vi "ControlRelay_ver10.vi"(0 "VISA session":refnum<visa-resource-name>="COM3", 1 "baud rate (9600)":u32=9600, 2 "data bits (8)":u16=8, 3 "stop bits (10: 1 bit)":u16(ring)=10 items=["1.0"=10, "1.5"=15, "2.0"=20], 4 "parity (0:none)":enum16{"None", "Odd", "Even", "Mark", "Space"}(ring), 5 "error in (no error)":errorcluster {"code" format="%.0x"}, 6 "BoardSelection":enum32{"Board A", "Board B"}(radio), 7 "Return Byte":u32=4, 8 "BoardA":T1(ring), 9 "flow control (0:none)":u16(ring) items=["None", "XON/XOFF", "RTS/CTS", "XON/XOFF & RTS/CTS", "DTR/DSR", "XON/XOFF & DTR/DSR"], 10 "BoardB":T2(ring), 11 "write buffer":string="Zc", 12 "Relay Setting":T3(radio)) -> (14 "Status of Set CMD":bool, 15 "ReturnCMD":string, 18 "Status of Manual CMD":bool, 19 "error out":errorcluster {"code" format="%.0x"})   [LabVIEW 2011]
uses:
  <vilib>/Instr/_visa.llb/VISA Configure Serial Port (Instr).vi
panel:
  out "read buffer 2":string
  out "after substring":string
  out "before substring":string
  out "TestPlanOutA":string caption="TestPlan on Board A"
  out "TestPlanOutB":string caption="TestPlan on Board B"
  in  "BoardB_TestPlan":T4(ring)
  in  "BoardA_TestPlan":T5(ring)
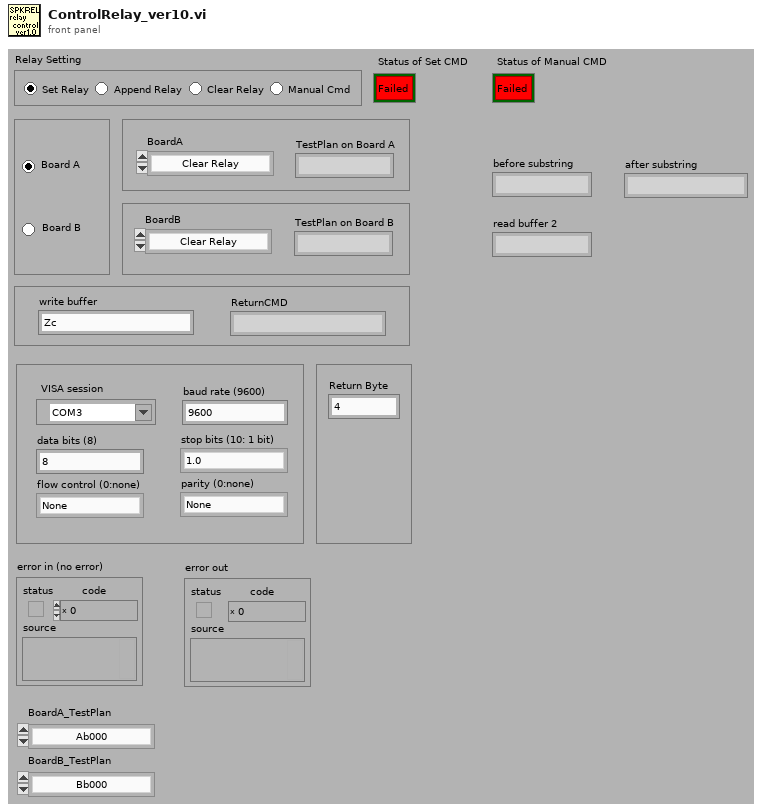
[diagram p1: front panel]
types:
  T1 = enum16{"Clear Relay", "Move Fixture in", "Move Fixture out", "Press UUT", "Press micro SW ", "Probe location M1", "Initial test 1", "Initial test 2", "Initial test 3", "Initial test 4", "Initial test 5", "Initial test 6", "Initial test 7", "Initial test 8", "Initial test 9", "Initial test 10", "Power on UUT", "Test of service pin", "Test of I2C Reset", "Test of I2C Address", "Test of I2C SDA", "Test of I2C SCK"}
  T2 = enum16{"Clear Relay", "Verify Fixture", "Connect RS 232 to UUT", "Test of CD Sinking", "Test of CTS Sinking", "Test of DTR Sinking", "Test of RTS", "Test of DSR", "Test of Lon bus (EKC204A1)", "Test of Lon bus CPU (SM Dummy )", "Test of RS485 (EKC204A2)", "Test of LAN Interface"}
  T3 = enum32{"Set Relay", "Append Relay", "Clear Relay", "Manual Cmd"}
  T4 = enum16{"Bb000", "Bb001", "Bb002", "Bb003", "Bb004", "Bb005", "Bb006", "Bb007", "Bb008", "Bb009", "Bb010", "Bb011"}
  T5 = enum16{"Ab000", "Ab001", "Ab002", "Ab003", "Ab004", "Ab005", "Ab006", "Ab007", "Ab008", "Ab009", "Ab010", "Ab011", "Ab012", "Ab013", "Ab014", "Ab015", "Ab016", "Ab017", "Ab018", "Ab019", "Ab020", "Ab021"}
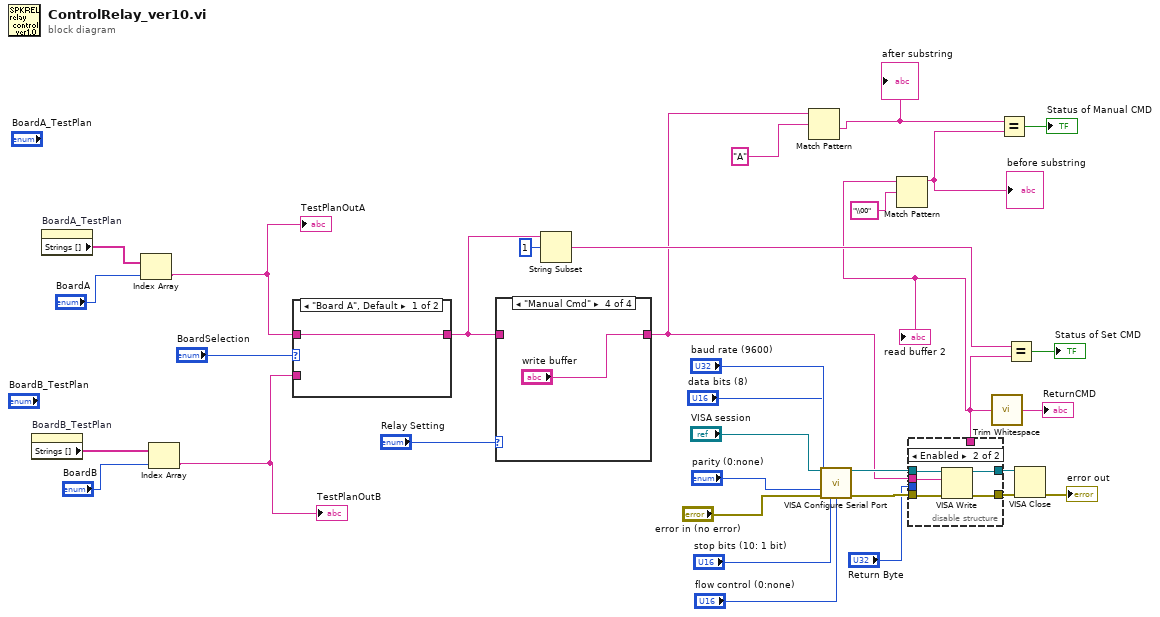
[diagram p0: block diagram]
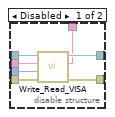
[diagram p2: hidden frame]
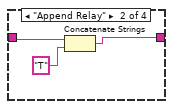
[diagram p4: hidden frame]
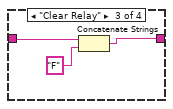
[diagram p5: hidden frame]
diagram:
  n1 = property on="BoardB_TestPlan" class="Enum (strict)"() -> ("Strings []"=w30:string[])  [unwired: 2 in, 2 out]
  n2 = property on="BoardA_TestPlan" class="Enum (strict)"() -> ("Strings []"=w31:string[])  [unwired: 2 in, 2 out]
  n3 = Index Array(array=w31, index="BoardA") -> (element=w8:string)
  "TestPlanOutA" <- w8
  n4 = Index Array(array=w30, index="BoardB") -> (element=w9:string)
  "TestPlanOutB" <- w9
  n5 = case shown="\"Board A\", Default" "BoardSelection" {
    tunnel: w8 -> [w34 _]
    tunnel: [w34 w35] -> w14
    tunnel: w9 -> [_ w35]
    frame "Board A", Default {
    }
    frame "Board B" {
    }
  }
  n6 = case shown="\"Manual Cmd\"" "Relay Setting" {
    tunnel: w14 -> [w36 w39 w41 _]
    tunnel: [w36 w38 w40 "write buffer"] -> w6
    frame "Set Relay", Default {
    }
    frame "Append Relay" {
      n7 = Concatenate Strings(w39, "T" ("string")) -> (w38:string)
    }
    frame "Clear Relay" {
      n8 = Concatenate Strings(w41, "F" ("string")) -> (w40:string)
    }
    frame "Manual Cmd" {
    }
  }
  n9 = String Subset(string=w14, offset (0)=1) -> (substring=w12:string)  [unwired: 1 out]
  n10 = Match Pattern(string=w6, regular expression="A") -> (after substring=w4:string)  [unwired: 4 out]
  "after substring" <- w4
  n11 = call-poly "VISA Configure Serial Port"("VISA resource name"="VISA session", "baud rate (9600)"="baud rate (9600)", "data bits (8)"="data bits (8)", "parity (0:none)"="parity (0:none)", "error in (no error)"="error in (no error)", "stop bits (10: 1 bit)"="stop bits (10: 1 bit)", "flow control (0:none)"="flow control (0:none)") -> ("VISA resource name out"=w23:refnum<visa-resource-name>, "error out"=w24:errorcluster)  [unwired: 7 out]
  n12 = disable-structure shown="Enabled" {
    disable-tunnel: [w50 w55] -> w26
    disable-tunnel: [w49 w51] -> w25
    disable-tunnel: w24 -> [w48 w54]
    disable-tunnel: w23 -> [w47 w53]
    disable-tunnel: "Return Byte" -> [w46 _]
    disable-tunnel: w6 -> [w45 w52]
    disable-tunnel: [w44 _] -> w3
    frame Disabled {
      n13 = call "Write_Read_VISA.vi"("error in (no error)"=w48, "Return Byte"=w46, "write buffer"=w45, "VISA session"=w47) -> ("error out"=w50:errorcluster, "read buffer"=w44:string, "dup VISA session"=w49:refnum<visa-resource-name>)  [unwired: 5 out]
    }
    frame Enabled {
      n14 = VISA Write(VISA resource name=w53, write buffer=w52, error in (no error)=w54) -> (VISA resource name out=w51:refnum<visa-resource-name>, error out=w55:errorcluster)  [unwired: 1 out]
    }
  }
  "read buffer 2" <- w3
  n15 = Match Pattern(string=w3, regular expression="\\00") -> (before substring=w1:string)  [unwired: 4 out]
  "before substring" <- w1
  n16 = call <vilib>:"Trim Whitespace.vi"("string"=w3) -> ("trimmed string"=→"ReturnCMD":string)  [unwired: 1 in]
  n17 = Equal?(x=w4, y=w1) -> (x = y?=→"Status of Manual CMD":bool)
  n18 = Equal?(x=w12, y=w3) -> (x = y?=→"Status of Set CMD":bool)
  n19 = VISA Close(VISA resource name=w25, error in (no error)=w26) -> (error out=→"error out":errorcluster)
